vi "Get Phase.vi"(6 "Output channel":i32, 8 "error in (no error)":errorcluster, 11 "RP Instrument in":refnum<class "RP Instrument.lvclass">) -> (0 "error out":errorcluster, 2 "Phase":u32=1 format="0x%x (%d)", 3 "RP Instrument out":refnum<class "RP Instrument.lvclass">)   [LabVIEW 2024, in "RP Instrument.lvclass"]
uses:
  RP Instrument.lvclass
  RP Instrument.lvclass/RP Instrument.ctl
  RP Communicator/RP Communicator.lvclass
  RP Status Offsets.ctl
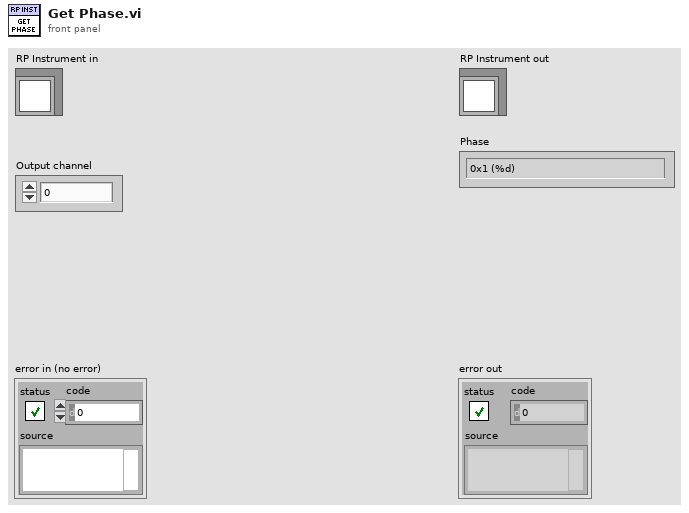
[diagram p1: front panel]
types:
  T1 = typedef "RP Status Offsets.ctl" = u16
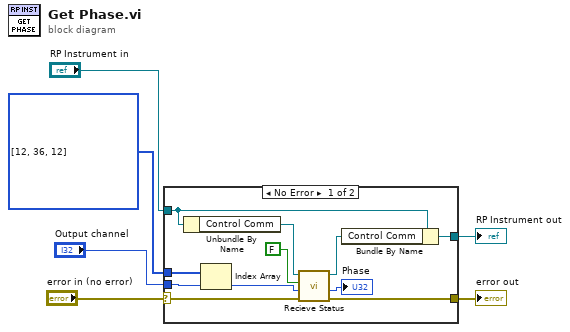
[diagram p0: block diagram]
diagram:
  w1 = T1[] [12, 36, 12] items=["Writer address"=0, "Record start position"=4, "Trig state and ID"=8, "Phase 0"=12, "X1"=16, "Y1"=20, "RxFIFO counter or  X2"=24, "TxFIFO counter or Y2"=28, "DDS modulus"=32, "Phase 1"=36]
  n1 = case shown="No Error" "error in (no error)" {
    selector: "error in (no error)" -> [w14 w19]
    tunnel: [w13 w19] -> w5
    tunnel: [w10 w18] -> w3
    tunnel: "RP Instrument in" -> [w11 w18]
    tunnel: "Output channel" -> [w8 _]
    tunnel: w1 -> [w7 _]
    frame No Error {
      n2 = Unbundle By Name(w11) -> ("Control Comm"=w17:refnum<class "RP Communicator.lvclass">)
      n3 = Index Array(array=w7, index=w8) -> (element=w9:T1)
      n4 = call-dynamic "Recieve Status.vi"("error in (no error)"=w14, "Status offset"=w9, "Read config instead"=FALSE, "RP Communicator in"=w17) -> ("error out"=w13:errorcluster, "Status response"=→"Phase":u32, "RP Communicator out"=w16:refnum<class "RP Communicator.lvclass">)  [unwired: 5 in]
      n5 = Bundle By Name(cluster=w11, "Control Comm"=w16) -> (w10:refnum<class "RP Instrument.lvclass">)
    }
    frame Error {
    }
  }
  "error out" <- w5
  "RP Instrument out" <- w3
